vi "Get Definition VIs Paths.vi"(8 "error in (no error)":errorcluster, 11 "owning references":T1) -> (0 "error out":errorcluster, 1 "Get Index Definition":path, 2 "Get Data Definition":path, 3 "owning references 2":T1)   [LabVIEW 2014, in "control module data interface generator.lvlib"]
uses:
  control module data interface generator.lvlib
  Controls/owning references.ctl
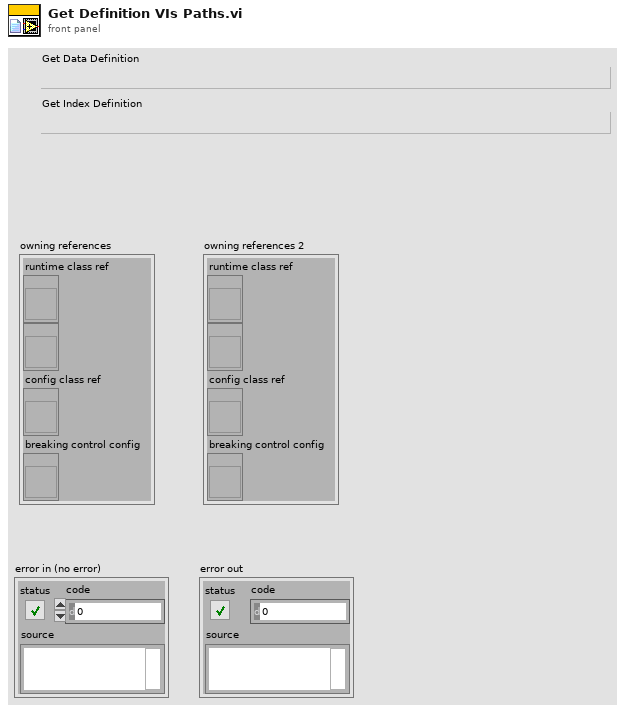
[diagram p1: front panel]
types:
  T1 = typedef "owning references.ctl" = cluster{"runtime class ref":refnum<vi>, "breaking control runtime":refnum<vi>, "config class ref":refnum<vi>, "breaking control config":refnum<vi>}
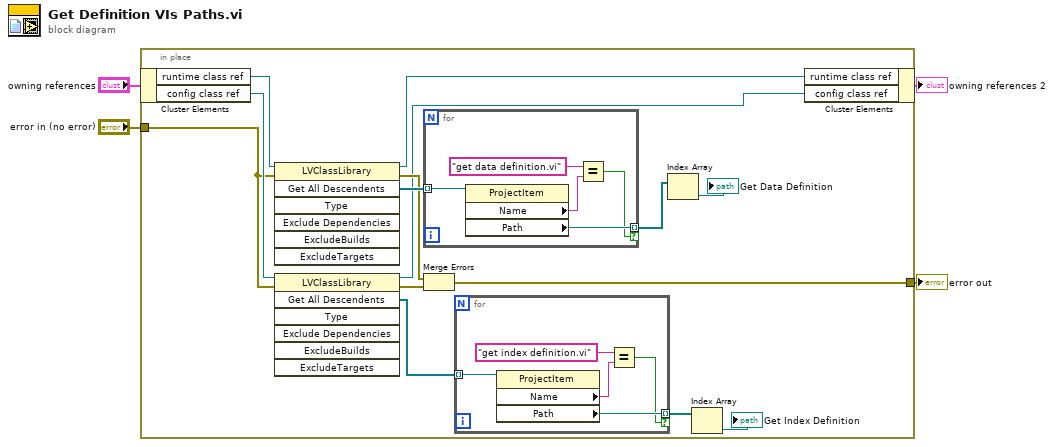
[diagram p0: block diagram]
diagram:
  n1 = in-place {
    in-place-border: "error in (no error)" -> [w10]
    in-place-border: [w12] -> w2
    n2 = in-place-cluster #1("owning references") -> ("runtime class ref"=w18:refnum<vi>, "config class ref"=w14:refnum<vi>)
    n3 = invoke class="LVClassLibrary" method="Get All Descendents"(reference=w18, error in=w10) -> (reference out=w16:refnum<vi>, error out=w15:errorcluster, "All Descendents"=w17:refnum<vi>[])  [unwired: 5 in, 4 out]
    n4 = invoke class="LVClassLibrary" method="Get All Descendents"(reference=w14, error in=w10) -> (reference out=w13:refnum<vi>, error out=w11:errorcluster, "All Descendents"=w7:refnum<vi>[])  [unwired: 5 in, 4 out]
    n5 = for {
      tunnel: w17 -> [w28] mode=indexing
      tunnel: [w27] -> w9 mode=indexing if=w24
      n6 = property class="ProjectItem"(reference=w28) -> ("Name"=w26:string, "Path"=w27:path)  [unwired: 1 in, 2 out]
      n7 = Equal?(x="get data definition.vi", y=w26) -> (x = y?=w24:bool)
    }
    n8 = Merge Errors(w15, w11) -> (w12:errorcluster)
    n9 = for {
      tunnel: w7 -> [w23] mode=indexing
      tunnel: [w22] -> w5 mode=indexing if=w19
      n10 = property class="ProjectItem"(reference=w23) -> ("Name"=w21:string, "Path"=w22:path)  [unwired: 1 in, 2 out]
      n11 = Equal?(x="get index definition.vi", y=w21) -> (x = y?=w19:bool)
    }
    n12 = Index Array(array=w9) -> (element=→"Get Data Definition":path)  [unwired: 1 in]
    n13 = Index Array(array=w5) -> (element=→"Get Index Definition":path)  [unwired: 1 in]
    n14 = in-place-cluster #1("runtime class ref"=w16, "config class ref"=w13) -> (→"owning references 2":T1)
  }
  "error out" <- w2
